vi "GeoData.vi"() -> ()   [LabVIEW 2017] (continued)
\tH1\n55474\t27053\tMinneapolis\tMN\tHennepin County\tH1\n55356\t27053\tLong lake\tMN\tHennepin County\tH1\n55404\t27053\tMinneapolis\tMN\tHennepin County\tH1\n55411\t27053\tMinneapolis\tMN\tHennepin County\tH1\n55423\t27053\tMinneapolis\tMN\tHennepin County\tH1\n55424\t27053\tMinneapolis\tMN\tHennepin County\tH1\n55429\t27053\tMinneapolis\tMN\tHennepin County\tH1\n55436\t27053\tMinneapolis\tMN\tHennepin County\tH1\n55420\t27053\tMinneapolis\tMN\tHennepin County\tH1\n55414\t27053\tMinneapolis\tMN\tHennepin County\tH1\n55416\t27053\tMinneapolis\tMN\tHennepin County\tH1\n55412\t27053\tMinneapolis\tMN\tHennepin County\tH1\n55419\t27053\tMinneapolis\tMN\tHennepin County\tH1\n55454\t27053\tMinneapolis\tMN\tHennepin County\tH1\n55442\t27053\tMinneapolis\tMN\tHennepin County\tH1\n55450\t27053\tMinneapolis\tMN\tHennepin County\tH1\n55480\t27053\tMinneapolis\tMN\tHennepin County\tH1\n55467\t27053\tMinneapolis\tMN\tHennepin County\tH1\n55305\t27053\tHopkins\tMN\tHennepin County\tH1\n55369\t27053\tOsseo\tMN\tHennepin County\tH1\n55391\t27053\tWayzata\tMN\tHennepin County\tH1\n55347\t27053\tEden prairie\tMN\tHennepin County\tH1\n55407\t27053\tMinneapolis\tMN\tHennepin County\tH1\n55357\t27053\tLoretto\tMN\tHennepin County\tH1\n55422\t27053\tMinneapolis\tMN\tHennepin County\tH1\n55427\t27053\tMinneapolis\tMN\tHennepin County\tH1\n55430\t27053\tMinneapolis\tMN\tHennepin County\tH1\n55415\t27053\tMinneapolis\tMN\tHennepin County\tH1\n55323\t27053\tCrystal bay\tMN\tHennepin County\tH1\n55488\t27053\tMinneapolis\tMN\tHennepin County\tH1\n55931\t27055\tEitzen\tMN\tHouston County\tH1\n55971\t27055\tRushford\tMN\tHouston County\tH1\n55947\t27055\tLa crescent\tMN\tHouston County\tH1\n55943\t27055\tHouston\tMN\tHouston County\tH1\n55921\t27055\tCaledonia\tMN\tHouston County\tH1\n55954\t27055\tMabel\tMN\tHouston County\tH1\n55974\t27055\tSpring grove\tMN\tHouston County\tH1\n55919\t27055\tBrownsville\tMN\tHouston County\tH1\n55941\t27055\tHokah\tMN\tHouston County\tH1\n56678\t27057\tSolway\tMN\tHubbard County\tH1\n56436\t27057\tBenedict\tMN\tHubbard County\tH1\n56464\t27057\tMenahga\tMN\tHubbard County\tH1\n56461\t27057\tLaporte\tMN\tHubbard County\tH1\n56633\t27057\tCass lake\tMN\tHubbard County\tH1\n56470\t27057\tPark rapids\tMN\tHubbard County\tH1\n56601\t27057\tBemidji\tMN\tHubbard County\tH1\n56467\t27057\tNevis\tMN\tHubbard County\tH1\n56458\t27057\tLake george\tMN\tHubbard County\tH1\n56484\t27057\tWalker\tMN\tHubbard County\tH1\n56433\t27057\tAkeley\tMN\tHubbard County\tH1\n56435\t27057\tBackus\tMN\tHubbard County\tH1\n56353\t27059\tMilaca\tMN\tIsanti County\tH1\n56358\t27059\tOgilvie\tMN\tIsanti County\tH1\n55032\t27059\tHarris\tMN\tIsanti County\tH1\n55017\t27059\tDalbo\tMN\tIsanti County\tH1\n55080\t27059\tStanchfield\tMN\tIsanti County\tH1\n55008\t27059\tCambridge\tMN\tIsanti County\tH1\n55006\t27059\tBraham\tMN\tIsanti County\tH1\n55056\t27059\tNorth branch\tMN\tIsanti County\tH1\n55070\t27059\tSaint francis\tMN\tIsanti County\tH1\n55398\t27059\tZimmerman\tMN\tIsanti County\tH1\n55029\t27059\tGrandy\tMN\tIsanti County\tH1\n55005\t27059\tBethel\tMN\tIsanti County\tH1\n55040\t27059\tIsanti\tMN\tIsanti County\tH1\n55079\t27059\tStacy\tMN\tIsanti County\tH1\n55371\t27059\tPrinceton\tMN\tIsanti County\tH1\n55771\t27061\tOrr\tMN\tItasca County\tH1\n56636\t27061\tDeer river\tMN\tItasca County\tH1\n55781\t27061\tSide lake\tMN\tItasca County\tH1\n55736\t27061\tFloodwood\tMN\tItasca County\tH1\n56630\t27061\tBlackduck\tMN\tItasca County\tH1\n56628\t27061\tBigfork\tMN\tItasca County\tH1\n56681\t27061\tSquaw lake\tMN\tItasca County\tH1\n55723\t27061\tCook\tMN\tItasca County\tH1\n55769\t27061\tNashwauk\tMN\tItasca County\tH1\n55709\t27061\tBovey\tMN\tItasca County\tH1\n56661\t27061\tNorthome\tMN\tItasca County\tH1\n56680\t27061\tSpring lake\tMN\tItasca County\tH1\n56639\t27061\tEffie\tMN\tItasca County\tH1\n55764\t27061\tMarble\tMN\tItasca County\tH1\n55753\t27061\tKeewatin\tMN\tItasca County\tH1\n55745\t27061\tGrand rapids\tMN\tItasca County\tH1\n55746\t27061\tHibbing\tMN\tItasca County\tH1\n55742\t27061\tGoodland\tMN\tItasca County\tH1\n55775\t27061\tPengilly\tMN\tItasca County\tH1\n56657\t27061\tMarcell\tMN\tItasca County\tH1\n56688\t27061\tWirt\tMN\tItasca County\tH1\n55744\t27061\tGrand rapids\tMN\tItasca County\tH1\n56659\t27061\tMax\tMN\tItasca County\tH1\n55722\t27061\tColeraine\tMN\tItasca County\tH1\n55752\t27061\tJacobson\tMN\tItasca County\tH1\n55793\t27061\tWarba\tMN\tItasca County\tH1\n56637\t27061\tTalmoon\tMN\tItasca County\tH1\n55748\t27061\tHill city\tMN\tItasca County\tH1\n55721\t27061\tCohasset\tMN\tItasca County\tH1\n55784\t27061\tSwan river\tMN\tItasca County\tH1\n55716\t27061\tCalumet\tMN\tItasca County\tH1\n56631\t27061\tBowstring\tMN\tItasca County\tH1\n55786\t27061\tTaconite\tMN\tItasca County\tH1\n56159\t27063\tMountain lake\tMN\tJackson County\tH1\n56160\t27063\tOdin\tMN\tJackson County\tH1\n56137\t27063\tHeron lake\tMN\tJackson County\tH1\n56150\t27063\tLakefield\tMN\tJackson County\tH1\n56187\t27063\tWorthington\tMN\tJackson County\tH1\n56143\t27063\tJackson\tMN\tJackson County\tH1\n56131\t27063\tFulda\tMN\tJackson County\tH1\n56119\t27063\tBrewster\tMN\tJackson County\tH1\n56167\t27063\tRound lake\tMN\tJackson County\tH1\n56111\t27063\tAlpha\tMN\tJackson County\tH1\n56101\t27063\tWindom\tMN\tJackson County\tH1\n56118\t27063\tBingham lake\tMN\tJackson County\tH1\n56161\t27063\tOkabena\tMN\tJackson County\tH1\n56127\t27063\tDunnell\tMN\tJackson County\tH1\n56353\t27065\tMilaca\tMN\tKanabec County\tH1\n56358\t27065\tOgilvie\tMN\tKanabec County\tH1\n55030\t27065\tGrasston\tMN\tKanabec County\tH1\n55037\t27065\tHinckley\tMN\tKanabec County\tH1\n56342\t27065\tIsle\tMN\tKanabec County\tH1\n55006\t27065\tBraham\tMN\tKanabec County\tH1\n55051\t27065\tMora\tMN\tKanabec County\tH1\n55007\t27065\tBrook park\tMN\tKanabec County\tH1\n55072\t27065\tSandstone\tMN\tKanabec County\tH1\n56312\t27067\tBelgrade\tMN\tKandiyohi County\tH1\n56201\t27067\tWillmar\tMN\tKandiyohi County\tH1\n56362\t27067\tPaynesville\tMN\tKandiyohi County\tH1\n56273\t27067\tNew london\tMN\tKandiyohi County\tH1\n56316\t27067\tBrooten\tMN\tKandiyohi County\tH1\n56284\t27067\tRenville\tMN\tKandiyohi County\tH1\n56289\t27067\tSunburg\tMN\tKandiyohi County\tH1\n56252\t27067\tKerkhoven\tMN\tKandiyohi County\tH1\n56281\t27067\tPrinsburg\tMN\tKandiyohi County\tH1\n56277\t27067\tOlivia\tMN\tKandiyohi County\tH1\n56288\t27067\tSpicer\tMN\tKandiyohi County\tH1\n56251\t27067\tKandiyohi\tMN\tKandiyohi County\tH1\n56216\t27067\tBlomkest\tMN\tKandiyohi County\tH1\n56253\t27067\tLake lillian\tMN\tKandiyohi County\tH1\n56243\t27067\tGrove city\tMN\tKandiyohi County\tH1\n56279\t27067\tPennock\tMN\tKandiyohi County\tH1\n56282\t27067\tRaymond\tMN\tKandiyohi County\tH1\n56222\t27067\tClara city\tMN\tKandiyohi County\tH1\n56209\t27067\tAtwater\tMN\tKandiyohi County\tH1\n56755\t27069\tSaint vincent\tMN\tKittson County\tH1\n56740\t27069\tNoyes\tMN\tKittson County\tH1\n56729\t27069\tHalma\tMN\tKittson County\tH1\n56733\t27069\tKennedy\tMN\tKittson County\tH1\n56734\t27069\tLake bronson\tMN\tKittson County\tH1\n56732\t27069\tKarlstad\tMN\tKittson County\tH1\n56731\t27069\tHumboldt\tMN\tKittson County\tH1\n56735\t27069\tLancaster\tMN\tKittson County\tH1\n56720\t27069\tDonaldson\tMN\tKittson County\tH1\n56728\t27069\tHallock\tMN\tKittson County\tH1\n55771\t27071\tOrr\tMN\tKoochiching County\tH1\n56654\t27071\tLoman\tMN\tKoochiching County\tH1\n56661\t27071\tNorthome\tMN\tKoochiching County\tH1\n56639\t27071\tEffie\tMN\tKoochiching County\tH1\n56668\t27071\tRanier\tMN\tKoochiching County\tH1\n56629\t27071\tBirchdale\tMN\tKoochiching County\tH1\n56660\t27071\tMizpah\tMN\tKoochiching County\tH1\n56653\t27071\tLittlefork\tMN\tKoochiching County\tH1\n56627\t27071\tBig falls\tMN\tKoochiching County\tH1\n56649\t27071\tInternational falls\tMN\tKoochiching County\tH1\n56679\t27071\tSouth international falls\tMN\tKoochiching County\tH1\n56623\t27071\tBaudette\tMN\tKoochiching County\tH1\n56669\t27071\tKabetogama\tMN\tKoochiching County\tH1\n56658\t27071\tMargie\tMN\tKoochiching County\tH1\n55772\t27071\tNett lake\tMN\tKoochiching County\tH1\n56223\t27073\tClarkfield\tMN\tLac qui Parle County\tH1\n56257\t27073\tMarietta\tMN\tLac qui Parle County\tH1\n56256\t27073\tMadison\tMN\tLac qui Parle County\tH1\n56278\t27073\tOrtonville\tMN\tLac qui Parle County\tH1\n56220\t27073\tCanby\tMN\tLac qui Parle County\tH1\n56265\t27073\tMontevideo\tMN\tLac qui Parle County\tH1\n56208\t27073\tAppleton\tMN\tLac qui Parle County\tH1\n56218\t27073\tBoyd\tMN\tLac qui Parle County\tH1\n56232\t27073\tDawson\tMN\tLac qui Parle County\tH1\n56276\t27073\tOdessa\tMN\tLac qui Parle County\tH1\n56212\t27073\tBellingham\tMN\tLac qui Parle County\tH1\n55614\t27075\tSilver bay\tMN\tLake County\tH1\n55616\t27075\tTwo harbors\tMN\tLake County\tH1\n55607\t27075\tIsabella\tMN\tLake County\tH1\n55731\t27075\tEly\tMN\tLake County\tH1\n55609\t27075\tKnife river\tMN\tLake County\tH1\n55602\t27075\tBrimson\tMN\tLake County\tH1\n55603\t27075\tFinland\tMN\tLake County\tH1\n55601\t27075\tBeaver bay\tMN\tLake County\tH1\n56711\t27077\tAngle inlet\tMN\tLake of the Woods County\tH1\n56623\t27077\tBaudette\tMN\tLake of the Woods County\tH1\n56673\t27077\tRoosevelt\tMN\tLake of the Woods County\tH1\n56741\t27077\tOak island\tMN\tLake of the Woods County\tH1\n56686\t27077\tWilliams\tMN\tLake of the Woods County\tH1\n56096\t27079\tWaterville\tMN\tLe Sueur County\tH1\n56052\t27079\tKilkenny\tMN\tLe Sueur County\tH1\n56050\t27079\tKasota\tMN\tLe Sueur County\tH1\n56071\t27079\tNew prague\tMN\tLe Sueur County\tH1\n56063\t27079\tMadison lake\tMN\tLe Sueur County\tH1\n56069\t27079\tMontgomery\tMN\tLe Sueur County\tH1\n56011\t27079\tBelle plaine\tMN\tLe Sueur County\tH1\n56058\t27079\tLe sueur\tMN\tLe Sueur County\tH1\n56057\t27079\tLe center\tMN\tLe Sueur County\tH1\n56028\t27079\tElysian\tMN\tLe Sueur County\tH1\n56082\t27079\tSaint peter\tMN\tLe Sueur County\tH1\n56017\t27079\tCleveland\tMN\tLe Sueur County\tH1\n56044\t27079\tHenderson\tMN\tLe Sueur County\tH1\n56264\t27081\tMinneota\tMN\tLincoln County\tH1\n56291\t27081\tTaunton\tMN\tLincoln County\tH1\n56170\t27081\tRuthton\tMN\tLincoln County\tH1\n56142\t27081\tIvanhoe\tMN\tLincoln County\tH1\n56178\t27081\tTyler\tMN\tLincoln County\tH1\n56220\t27081\tCanby\tMN\tLincoln County\tH1\n56136\t27081\tHendricks\tMN\tLincoln County\tH1\n56164\t27081\tPipestone\tMN\tLincoln County\tH1\n56113\t27081\tArco\tMN\tLincoln County\tH1\n56149\t27081\tLake benton\tMN\tLincoln County\tH1\n56280\t27081\tPorter\tMN\tLincoln County\tH1\n56264\t27083\tMinneota\tMN\tLyon County\tH1\n56291\t27083\tTaunton\tMN\tLyon County\tH1\n56170\t27083\tRuthton\tMN\tLyon County\tH1\n56157\t27083\tLynd\tMN\tLyon County\tH1\n56115\t27083\tBalaton\tMN\tLyon County\tH1\n56175\t27083\tTracy\tMN\tLyon County\tH1\n56178\t27083\tTyler\tMN\tLyon County\tH1\n56263\t27083\tMilroy\tMN\tLyon County\tH1\n56220\t27083\tCanby\tMN\tLyon County\tH1\n56258\t27083\tMarshall\tMN\tLyon County\tH1\n56297\t27083\tWood lake\tMN\tLyon County\tH1\n56229\t27083\tCottonwood\tMN\tLyon County\tH1\n56239\t27083\tGhent\tMN\tLyon County\tH1\n56113\t27083\tArco\tMN\tLyon County\tH1\n56169\t27083\tRussell\tMN\tLyon County\tH1\n56132\t27083\tGarvin\tMN\tLyon County\tH1\n56280\t27083\tPorter\tMN\tLyon County\tH1\n55312\t27085\tBrownton\tMN\tMcLeod County\tH1\n55370\t27085\tPlato\tMN\tMcLeod County\tH1\n55355\t27085\tLitchfield\tMN\tMcLeod County\tH1\n55368\t27085\tNorwood young america\tMN\tMcLeod County\tH1\n55339\t27085\tHamburg\tMN\tMcLeod County\tH1\n55350\t27085\tHutchinson\tMN\tMcLeod County\tH1\n55338\t27085\tGreen isle\tMN\tMcLeod County\tH1\n55381\t27085\tSilver lake\tMN\tMcLeod County\tH1\n55335\t27085\tGibbon\tMN\tMcLeod County\tH1\n55336\t27085\tGlencoe\tMN\tMcLeod County\tH1\n55354\t27085\tLester prairie\tMN\tMcLeod County\tH1\n55367\t27085\tNew germany\tMN\tMcLeod County\tH1\n55396\t27085\tWinthrop\tMN\tMcLeod County\tH1\n55385\t27085\tStewart\tMN\tMcLeod County\tH1\n55397\t27085\tYoung america\tMN\tMcLeod County\tH1\n55395\t27085\tWinsted\tMN\tMcLeod County\tH1\n56651\t27087\tLengby\tMN\tMahnomen County\tH1\n56621\t27087\tBagley\tMN\tMahnomen County\tH1\n56540\t27087\tFertile\tMN\tMahnomen County\tH1\n56589\t27087\tWaubun\tMN\tMahnomen County\tH1\n56592\t27087\tWinger\tMN\tMahnomen County\tH1\n56566\t27087\tNaytahwaush\tMN\tMahnomen County\tH1\n56557\t27087\tMahnomen\tMN\tMahnomen County\tH1\n56542\t27087\tFosston\tMN\tMahnomen County\tH1\n56516\t27087\tBejou\tMN\tMahnomen County\tH1\n56727\t27089\tGrygla\tMN\tMarshall County\tH1\n56744\t27089\tOslo\tMN\tMarshall County\tH1\n56757\t27089\tStephen\tMN\tMarshall County\tH1\n56762\t27089\tWarren\tMN\tMarshall County\tH1\n56724\t27089\tGatzke\tMN\tMarshall County\tH1\n56758\t27089\tStrandquist\tMN\tMarshall County\tH1\n56760\t27089\tViking\tMN\tMarshall County\tH1\n56738\t27089\tNewfolden\tMN\tMarshall County\tH1\n56732\t27089\tKarlstad\tMN\tMarshall County\tH1\n56759\t27089\tStrathcona\tMN\tMarshall County\tH1\n56710\t27089\tAlvarado\tMN\tMarshall County\tH1\n56701\t27089\tThief river falls\tMN\tMarshall County\tH1\n56713\t27089\tArgyle\tMN\tMarshall County\tH1\n56725\t27089\tGoodridge\tMN\tMarshall County\tH1\n56737\t27089\tMiddle river\tMN\tMarshall County\tH1\n56098\t27091\tWinnebago\tMN\tMartin County\tH1\n56027\t27091\tElmore\tMN\tMartin County\tH1\n56162\t27091\tOrmsby\tMN\tMartin County\tH1\n56160\t27091\tOdin\tMN\tMartin County\tH1\n56031\t27091\tFairmont\tMN\tMartin County\tH1\n56181\t27091\tWelcome\tMN\tMartin County\tH1\n56075\t27091\tNorthrop\tMN\tMartin County\tH1\n56176\t27091\tTrimont\tMN\tMartin County\tH1\n56171\t27091\tSherburn\tMN\tMartin County\tH1\n56121\t27091\tCeylon\tMN\tMartin County\tH1\n56013\t27091\tBlue earth\tMN\tMartin County\tH1\n56111\t27091\tAlpha\tMN\tMartin County\tH1\n56039\t27091\tGranada\tMN\tMartin County\tH1\n56088\t27091\tTruman\tMN\tMartin County\tH1\n56127\t27091\tDunnell\tMN\tMartin County\tH1\n55353\t27093\tKimball\tMN\tMeeker County\tH1\n56362\t27093\tPaynesville\tMN\tMeeker County\tH1\n56228\t27093\tCosmos\tMN\tMeeker County\tH1\n55324\t27093\tDarwin\tMN\tMeeker County\tH1\n55355\t27093\tLitchfield\tMN\tMeeker County\tH1\n55389\t27093\tWatkins\tMN\tMeeker County\tH1\n55350\t27093\tHutchinson\tMN\tMeeker County\tH1\n55321\t27093\tCokato\tMN\tMeeker County\tH1\n55342\t27093\tHector\tMN\tMeeker County\tH1\n55382\t27093\tSouth haven\tMN\tMeeker County\tH1\n55329\t27093\tEden valley\tMN\tMeeker County\tH1\n56243\t27093\tGrove city\tMN\tMeeker County\tH1\n55325\t27093\tDassel\tMN\tMeeker County\tH1\n56209\t27093\tAtwater\tMN\tMeeker County\tH1\n56353\t27095\tMilaca\tMN\tMille Lacs County\tH1\n56358\t27095\tOgilvie\tMN\tMille Lacs County\tH1\n56363\t27095\tPease\tMN\tMille Lacs County\tH1\n56313\t27095\tBock\tMN\tMille Lacs County\tH1\n56330\t27095\tForeston\tMN\tMille Lacs County\tH1\n56342\t27095\tIsle\tMN\tMille Lacs County\tH1\n56338\t27095\tHillman\tMN\tMille Lacs County\tH1\n56359\t27095\tOnamia\tMN\tMille Lacs County\tH1\n56450\t27095\tGarrison\tMN\tMille Lacs County\tH1\n55371\t27095\tPrinceton\tMN\tMille Lacs County\tH1\n56357\t27095\tOak park\tMN\tMille Lacs County\tH1\n56386\t27095\tWahkon\tMN\tMille Lacs County\tH1\n56353\t27097\tMilaca\tMN\tMorrison County\tH1\n56364\t27097\tPierz\tMN\tMorrison County\tH1\n56347\t27097\tLong prairie\tMN\tMorrison County\tH1\n56307\t27097\tAlbany\tMN\tMorrison County\tH1\n56345\t27097\tLittle falls\tMN\tMorrison County\tH1\n56336\t27097\tGrey eagle\tMN\tMorrison County\tH1\n56443\t27097\tCushing\tMN\tMorrison County\tH1\n56314\t27097\tBowlus\tMN\tMorrison County\tH1\n56338\t27097\tHillman\tMN\tMorrison County\tH1\n56367\t27097\tRice\tMN\tMorrison County\tH1\n56331\t27097\tFreeport\tMN\tMorrison County\tH1\n56328\t27097\tFlensburg\tMN\tMorrison County\tH1\n56384\t27097\tUpsala\tMN\tMorrison County\tH1\n56344\t27097\tLastrup\tMN\tMorrison County\tH1\n56318\t27097\tBurtrum\tMN\tMorrison County\tH1\n56359\t27097\tOnamia\tMN\tMorrison County\tH1\n56473\t27097\tPillager\tMN\tMorrison County\tH1\n56449\t27097\tFort ripley\tMN\tMorrison County\tH1\n56466\t27097\tMotley\tMN\tMorrison County\tH1\n56373\t27097\tRoyalton\tMN\tMorrison County\tH1\n56340\t27097\tHoldingford\tMN\tMorrison County\tH1\n56475\t27097\tRandall\tMN\tMorrison County\tH1\n56329\t27097\tFoley\tMN\tMorrison County\tH1\n56382\t27097\tSwanville\tMN\tMorrison County\tH1\n55926\t27099\tDexter\tMN\tMower County\tH1\n55936\t27099\tGrand meadow\tMN\tMower County\tH1\n55975\t27099\tSpring valley\tMN\tMower County\tH1\n55918\t27099\tBrownsdale\tMN\tMower County\tH1\n55951\t27099\tLe roy\tMN\tMower County\tH1\n55917\t27099\tBlooming prairie\tMN\tMower County\tH1\n55909\t27099\tAdams\tMN\tMower County\tH1\n55967\t27099\tRacine\tMN\tMower County\tH1\n55933\t27099\tElkton\tMN\tMower County\tH1\n55973\t27099\tSargeant\tMN\tMower County\tH1\n55940\t27099\tHayfield\tMN\tMower County\tH1\n55976\t27099\tStewartville\tMN\tMower County\tH1\n55970\t27099\tRose creek\tMN\tMower County\tH1\n55950\t27099\tLansing\tMN\tMower County\tH1\n55912\t27099\tAustin\tMN\tMower County\tH1\n55961\t27099\tOstrander\tMN\tMower County\tH1\n55982\t27099\tWaltham\tMN\tMower County\tH1\n55953\t27099\tLyle\tMN\tMower County\tH1\n55977\t27099\tTaopi\tMN\tMower County\tH1\n56180\t27101\tWalnut grove\tMN\tMurray County\tH1\n56172\t27101\tSlayton\tMN\tMurray County\tH1\n56170\t27101\tRuthton\tMN\tMurray County\tH1\n56141\t27101\tIona\tMN\tMurray County\tH1\n56125\t27101\tDovray\tMN\tMurray County\tH1\n56115\t27101\tBalaton\tMN\tMurray County\tH1\n56122\t27101\tChandler\tMN\tMurray County\tH1\n56151\t27101\tLake wilson\tMN\tMurray County\tH1\n56175\t27101\tTracy\tMN\tMurray County\tH1\n56114\t27101\tAvoca\tMN\tMurray County\tH1\n56131\t27101\tFulda\tMN\tMurray County\tH1\n56186\t27101\tWoodstock\tMN\tMurray County\tH1\n56128\t27101\tEdgerton\tMN\tMurray County\tH1\n56183\t27101\tWestbrook\tMN\tMurray County\tH1\n56123\t27101\tCurrie\tMN\tMurray County\tH1\n56132\t27101\tGarvin\tMN\tMurray County\tH1\n56149\t27101\tLake benton\tMN\tMurray County\tH1\n56054\t27103\tLafayette\tMN\tNicollet County\tH1\n55335\t27103\tGibbon\tMN\tNicollet County\tH1\n56001\t27103\tMankato\tMN\tNicollet County\tH1\n56058\t27103\tLe sueur\tMN\tNicollet County\tH1\n56003\t27103\tMankato\tMN\tNicollet County\tH1\n56073\t27103\tNew ulm\tMN\tNicollet County\tH1\n56074\t27103\tNicollet\tMN\tNicollet County\tH1\n55334\t27103\tGaylord\tMN\tNicollet County\tH1\n55332\t27103\tFairfax\tMN\tNicollet County\tH1\n56082\t27103\tSaint peter\tMN\tNicollet County\tH1\n56021\t27103\tCourtland\tMN\tNicollet County\tH1\n56158\t27105\tMagnolia\tMN\tNobles County\tH1\n56141\t27105\tIona\tMN\tNobles County\tH1\n56122\t27105\tChandler\tMN\tNobles County\tH1\n56137\t27105\tHeron lake\tMN\tNobles County\tH1\n56153\t27105\tLeota\tMN\tNobles County\tH1\n56110\t27105\tAdrian\tMN\tNobles County\tH1\n56187\t27105\tWorthington\tMN\tNobles County\tH1\n56131\t27105\tFulda\tMN\tNobles County\tH1\n56119\t27105\tBrewster\tMN\tNobles County\tH1\n56185\t27105\tWilmont\tMN\tNobles County\tH1\n56167\t27105\tRound lake\tMN\tNobles County\tH1\n56128\t27105\tEdgerton\tMN\tNobles County\tH1\n56165\t27105\tReading\tMN\tNobles County\tH1\n56117\t27105\tBigelow\tMN\tNobles County\tH1\n56129\t27105\tEllsworth\tMN\tNobles County\tH1\n56155\t27105\tLismore\tMN\tNobles County\tH1\n56168\t27105\tRushmore\tMN\tNobles County\tH1\n56147\t27105\tKenneth\tMN\tNobles County\tH1\n56584\t27107\tTwin valley\tMN\tNorman County\tH1\n56545\t27107\tGary\tMN\tNorman County\tH1\n56550\t27107\tHendrum\tMN\tNorman County\tH1\n56585\t27107\tUlen\tMN\tNorman County\tH1\n56541\t27107\tFlom\tMN\tNorman County\tH1\n56510\t27107\tAda\tMN\tNorman County\tH1\n56581\t27107\tShelly\tMN\tNorman County\tH1\n56574\t27107\tPerley\tMN\tNorman County\tH1\n56540\t27107\tFertile\tMN\tNorman County\tH1\n56589\t27107\tWaubun\tMN\tNorman County\tH1\n56546\t27107\tGeorgetown\tMN\tNorman County\tH1\n56519\t27107\tBorup\tMN\tNorman County\tH1\n56557\t27107\tMahnomen\tMN\tNorman County\tH1\n56568\t27107\tNielsville\tMN\tNorman County\tH1\n56548\t27107\tHalstad\tMN\tNorman County\tH1\n56516\t27107\tBejou\tMN\tNorman County\tH1\n55906\t27109\tRochester\tMN\tOlmsted County\tH1\n55960\t27109\tOronoco\tMN\tOlmsted County\tH1\n55944\t27109\tKasson\tMN\tOlmsted County\tH1\n55903\t27109\tRochester\tMN\tOlmsted County\tH1\n55901\t27109\tRochester\tMN\tOlmsted County\tH1\n55904\t27109\tRochester\tMN\tOlmsted County\tH1\n55923\t27109\tChatfield\tMN\tOlmsted County\tH1\n55905\t27109\tRochester\tMN\tOlmsted County\tH1\n55934\t27109\tEyota\tMN\tOlmsted County\tH1\n55955\t27109\tMantorville\tMN\tOlmsted County\tH1\n55920\t27109\tByron\tMN\tOlmsted County\tH1\n55972\t27109\tSaint charles\tMN\tOlmsted County\tH1\n55991\t27109\tZumbro falls\tMN\tOlmsted County\tH1\n55932\t27109\tElgin\tMN\tOlmsted County\tH1\n55973\t27109\tSargeant\tMN\tOlmsted County\tH1\n55902\t27109\tRochester\tMN\tOlmsted County\tH1\n55956\t27109\tMazeppa\tMN\tOlmsted County\tH1\n55940\t27109\tHayfield\tMN\tOlmsted County\tH1\n55964\t27109\tPlainview\tMN\tOlmsted County\tH1\n55963\t27109\tPine island\tMN\tOlmsted County\tH1\n55976\t27109\tStewartville\tMN\tOlmsted County\tH1\n55929\t27109\tDover\tMN\tOlmsted County\tH1\n56527\t27111\tDeer creek\tMN\tOtter Tail County\tH1\n56573\t27111\tPerham\tMN\tOtter Tail County\tH1\n56531\t27111\tElbow lake\tMN\tOtter Tail County\tH1\n56534\t27111\tErhard\tMN\tOtter Tail County\tH1\n56551\t27111\tHenning\tMN\tOtter Tail County\tH1\n56464\t27111\tMenahga\tMN\tOtter Tail County\tH1\n56315\t27111\tBrandon\tMN\tOtter Tail County\tH1\n56437\t27111\tBertha\tMN\tOtter Tail County\tH1\n56587\t27111\tVergas\tMN\tOtter Tail County\tH1\n56588\t27111\tVining\tMN\tOtter Tail County\tH1\n56567\t27111\tNew york mills\tMN\tOtter Tail County\tH1\n56528\t27111\tDent\tMN\tOtter Tail County\tH1\n56524\t27111\tClitherall\tMN\tOtter Tail County\tH1\n56477\t27111\tSebeka\tMN\tOtter Tail County\tH1\n56453\t27111\tHewitt\tMN\tOtter Tail County\tH1\n56590\t27111\tWendell\tMN\tOtter Tail County\tH1\n56309\t27111\tAshby\tMN\tOtter Tail County\tH1\n56361\t27111\tParkers prairie\tMN\tOtter Tail County\tH1\n56515\t27111\tBattle lake\tMN\tOtter Tail County\tH1\n56326\t27111\tEvansville\tMN\tOtter Tail County\tH1\n56533\t27111\tElizabeth\tMN\tOtter Tail County\tH1\n56579\t27111\tRothsay\tMN\tOtter Tail County\tH1\n56583\t27111\tTintah\tMN\tOtter Tail County\tH1\n56522\t27111\tCampbell\tMN\tOtter Tail County\tH1\n56324\t27111\tDalton\tMN\tOtter Tail County\tH1\n56514\t27111\tBarnesville\tMN\tOtter Tail County\tH1\n56572\t27111\tPelican rapids\tMN\tOtter Tail County\tH1\n56482\t27111\tWadena\tMN\tOtter Tail County\tH1\n56571\t27111\tOttertail\tMN\tOtter Tail County\tH1\n56354\t27111\tMiltona\tMN\tOtter Tail County\tH1\n56501\t27111\tDetroit lakes\tMN\tOtter Tail County\tH1\n56576\t27111\tRichville\tMN\tOtter Tail County\tH1\n56446\t27111\tEagle bend\tMN\tOtter Tail County\tH1\n56544\t27111\tFrazee\tMN\tOtter Tail County\tH1\n56537\t27111\tFergus falls\tMN\tOtter Tail County\tH1\n56586\t27111\tUnderwood\tMN\tOtter Tail County\tH1\n56518\t27111\tBluffton\tMN\tOtter Tail County\tH1\n56748\t27113\tPlummer\tMN\tPennington County\tH1\n56760\t27113\tViking\tMN\tPennington County\tH1\n56754\t27113\tSaint hilaire\tMN\tPennington County\tH1\n56750\t27113\tRed lake falls\tMN\tPennington County\tH1\n56701\t27113\tThief river falls\tMN\tPennington County\tH1\n56725\t27113\tGoodridge\tMN\tPennington County\tH1\n55063\t27115\tPine city\tMN\tPine County\tH1\n55069\t27115\tRush city\tMN\tPine County\tH1\n55036\t27115\tHenriette\tMN\tPine County\tH1\n55735\t27115\tFinlayson\tMN\tPine County\tH1\n55030\t27115\tGrasston\tMN\tPine County\tH1\n55037\t27115\tHinckley\tMN\tPine County\tH1\n55795\t27115\tWillow river\tMN\tPine County\tH1\n55749\t27115\tHolyoke\tMN\tPine County\tH1\n55756\t27115\tKerrick\tMN\tPine County\tH1\n55006\t27115\tBraham\tMN\tPine County\tH1\n56350\t27115\tMc grath\tMN\tPine County\tH1\n55051\t27115\tMora\tMN\tPine County\tH1\n55712\t27115\tBruno\tMN\tPine County\tH1\n55767\t27115\tMoose lake\tMN\tPine County\tH1\n55007\t27115\tBrook park\tMN\tPine County\tH1\n55072\t27115\tSandstone\tMN\tPine County\tH1\n55704\t27115\tAskov\tMN\tPine County\tH1\n55783\t27115\tSturgeon lake\tMN\tPine County\tH1\n56170\t27117\tRuthton\tMN\tPipestone County\tH1\n56164\t27117\tPipestone\tMN\tPipestone County\tH1\n56186\t27117\tWoodstock\tMN\tPipestone County\tH1\n56128\t27117\tEdgerton\tMN\tPipestone County\tH1\n56139\t27117\tHolland\tMN\tPipestone County\tH1\n56144\t27117\tJasper\tMN\tPipestone County\tH1\n56156\t27117\tLuverne\tMN\tPipestone County\tH1\n56149\t27117\tLake benton\tMN\tPipestone County\tH1\n56721\t27119\tEast grand forks\tMN\tPolk County\tH1\n56723\t27119\tFisher\tMN\tPolk County\tH1\n56556\t27119\tMcintosh\tMN\tPolk County\tH1\n56523\t27119\tClimax\tMN\tPolk County\tH1\n56744\t27119\tOslo\tMN\tPolk County\tH1\n56742\t27119\tOklee\tMN\tPolk County\tH1\n56651\t27119\tLengby\tMN\tPolk County\tH1\n56716\t27119\tCrookston\tMN\tPolk County\tH1\n56762\t27119\tWarren\tMN\tPolk County\tH1\n56621\t27119\tBagley\tMN\tPolk County\tH1\n56535\t27119\tErskine\tMN\tPolk County\tH1\n56722\t27119\tEuclid\tMN\tPolk County\tH1\n56540\t27119\tFertile\tMN\tPolk County\tH1\n56684\t27119\tTrail\tMN\tPolk County\tH1\n56592\t27119\tWinger\tMN\tPolk County\tH1\n56646\t27119\tGully\tMN\tPolk County\tH1\n56644\t27119\tGonvick\tMN\tPolk County\tH1\n56568\t27119\tNielsville\tMN\tPolk County\tH1\n56710\t27119\tAlvarado\tMN\tPolk County\tH1\n56542\t27119\tFosston\tMN\tPolk County\tH1\n56750\t27119\tRed lake falls\tMN\tPolk County\tH1\n56517\t27119\tBeltrami\tMN\tPolk County\tH1\n56736\t27119\tMentor\tMN\tPolk County\tH1\n56226\t27121\tClontarf\tMN\tPope County\tH1\n56323\t27121\tCyrus\tMN\tPope County\tH1\n56316\t27121\tBrooten\tMN\tPope County\tH1\n56343\t27121\tKensington\tMN\tPope County\tH1\n56349\t27121\tLowry\tMN\tPope County\tH1\n56289\t27121\tSunburg\tMN\tPope County\tH1\n56334\t27121\tGlenwood\tMN\tPope County\tH1\n56308\t27121\tAlexandria\tMN\tPope County\tH1\n56360\t27121\tOsakis\tMN\tPope County\tH1\n56378\t27121\tSauk centre\tMN\tPope County\tH1\n56215\t27121\tBenson\tMN\tPope County\tH1\n56381\t27121\tStarbuck\tMN\tPope County\tH1\n56327\t27121\tFarwell\tMN\tPope County\tH1\n56244\t27121\tHancock\tMN\tPope County\tH1\n56385\t27121\tVillard\tMN\tPope County\tH1\n55106\t27123\tSaint paul\tMN\tRamsey County\tH1\n55107\t27123\tSaint paul\tMN\tRamsey County\tH1\n55113\t27123\tSaint paul\tMN\tRamsey County\tH1\n55117\t27123\tSaint paul\tMN\tRamsey County\tH1\n55126\t27123\tSaint paul\tMN\tRamsey County\tH1\n55102\t27123\tSaint paul\tMN\tRamsey County\tH1\n55105\t27123\tSaint paul\tMN\tRamsey County\tH1\n55112\t27123\tSaint paul\tMN\tRamsey County\tH1\n55119\t27123\tSaint paul\tMN\tRamsey County\tH1\n55418\t27123\tMinneapolis\tMN\tRamsey County\tH1\n55104\t27123\tSaint paul\tMN\tRamsey County\tH1\n55108\t27123\tSaint paul\tMN\tRamsey County\tH1\n55114\t27123\tSaint paul\tMN\tRamsey County\tH1\n55118\t27123\tSaint paul\tMN\tRamsey County\tH1\n55127\t27123\tSaint paul\tMN\tRamsey County\tH1\n55449\t27123\tMinneapolis\tMN\tRamsey County\tH1\n55155\t27123\tSaint paul\tMN\tRamsey County\tH1\n55109\t27123\tSaint paul\tMN\tRamsey County\tH1\n55125\t27123\tSaint paul\tMN\tRamsey County\tH1\n55432\t27123\tMinneapolis\tMN\tRamsey County\tH1\n55146\t27123\tSaint paul\tMN\tRamsey County\tH1\n55421\t27123\tMinneapolis\tMN\tRamsey County\tH1\n55101\t27123\tSaint paul\tMN\tRamsey County\tH1\n55103\t27123\tSaint paul\tMN\tRamsey County\tH1\n55130\t27123\tSaint paul\tMN\tRamsey County\tH1\n55144\t27123\tSaint paul\tMN\tRamsey County\tH1\n55110\t27123\tSaint paul\tMN\tRamsey County\tH1\n55116\t27123\tSaint paul\tMN\tRamsey County\tH1\n55128\t27123\tSaint paul\tMN\tRamsey County\tH1\n56742\t27125\tOklee\tMN\tRed Lake County\tH1\n56716\t27125\tCrookston\tMN\tRed Lake County\tH1\n56748\t27125\tPlummer\tMN\tRed Lake County\tH1\n56535\t27125\tErskine\tMN\tRed Lake County\tH1\n56754\t27125\tSaint hilaire\tMN\tRed Lake County\tH1\n56715\t27125\tBrooks\tMN\tRed Lake County\tH1\n56750\t27125\tRed lake falls\tMN\tRed Lake County\tH1\n56736\t27125\tMentor\tMN\tRed Lake County\tH1\n56180\t27127\tWalnut grove\tMN\tRedwood County\tH1\n55333\t27127\tFranklin\tMN\tRedwood County\tH1\n56255\t27127\tLucan\tMN\tRedwood County\tH1\n56166\t27127\tRevere\tMN\tRedwood County\tH1\n56284\t27127\tRenville\tMN\tRedwood County\tH1\n56175\t27127\tTracy\tMN\tRedwood County\tH1\n56263\t27127\tMilroy\tMN\tRedwood County\tH1\n56266\t27127\tMorgan\tMN\tRedwood County\tH1\n56294\t27127\tWanda\tMN\tRedwood County\tH1\n56283\t27127\tRedwood falls\tMN\tRedwood County\tH1\n56258\t27127\tMarshall\tMN\tRedwood County\tH1\n56292\t27127\tVesta\tMN\tRedwood County\tH1\n56224\t27127\tClements\tMN\tRedwood County\tH1\n56214\t27127\tBelview\tMN\tRedwood County\tH1\n56085\t27127\tSleepy eye\tMN\tRedwood County\tH1\n56152\t27127\tLamberton\tMN\tRedwood County\tH1\n56297\t27127\tWood lake\tMN\tRedwood County\tH1\n56270\t27127\tMorton\tMN\tRedwood County\tH1\n56087\t27127\tSpringfield\tMN\tRedwood County\tH1\n56287\t27127\tSeaforth\tMN\tRedwood County\tH1\n56237\t27127\tEcho\tMN\tRedwood County\tH1\n56083\t27127\tSanborn\tMN\tRedwood County\tH1\n56293\t27127\tWabasso\tMN\tRedwood County\tH1\n55310\t27129\tBird island\tMN\tRenville County\tH1\n55333\t27129\tFranklin\tMN\tRenville County\tH1\n56228\t27129\tCosmos\tMN\tRenville County\tH1\n56241\t27129\tGranite falls\tMN\tRenville County\tH1\n56284\t27129\tRenville\tMN\tRenville County\tH1\n55350\t27129\tHutchinson\tMN\tRenville County\tH1\n55342\t27129\tHector\tMN\tRenville County\tH1\n56277\t27129\tOlivia\tMN\tRenville County\tH1\n56283\t27129\tRedwood falls\tMN\tRenville County\tH1\n56260\t27129\tMaynard\tMN\tRenville County\tH1\n56285\t27129\tSacred heart\tMN\tRenville County\tH1\n56270\t27129\tMorton\tMN\tRenville County\tH1\n56230\t27129\tDanube\tMN\tRenville County\tH1\n55385\t27129\tStewart\tMN\tRenville County\tH1\n55332\t27129\tFairfax\tMN\tRenville County\tH1\n55314\t27129\tBuffalo lake\tMN\tRenville County\tH1\n56096\t27131\tWaterville\tMN\tRice County\tH1\n55049\t27131\tMedford\tMN\tRice County\tH1\n55946\t27131\tKenyon\tMN\tRice County\tH1\n56052\t27131\tKilkenny\tMN\tRice County\tH1\n55057\t27131\tNorthfield\tMN\tRice County\tH1\n55020\t27131\tElko new market\tMN\tRice County\tH1\n55046\t27131\tLonsdale\tMN\tRice County\tH1\n56071\t27131\tNew prague\tMN\tRice County\tH1\n55019\t27131\tDundas\tMN\tRice County\tH1\n56069\t27131\tMontgomery\tMN\tRice County\tH1\n55088\t27131\tWebster\tMN\tRice County\tH1\n55021\t27131\tFaribault\tMN\tRice County\tH1\n55018\t27131\tDennison\tMN\tRice County\tH1\n55087\t27131\tWarsaw\tMN\tRice County\tH1\n55053\t27131\tNerstrand\tMN\tRice County\tH1\n55052\t27131\tMorristown\tMN\tRice County\tH1\n56158\t27133\tMagnolia\tMN\tRock County\tH1\n56173\t27133\tSteen\tMN\tRock County\tH1\n56146\t27133\tKanaranzi\tMN\tRock County\tH1\n56134\t27133\tHardwick\tMN\tRock County\tH1\n56116\t27133\tBeaver creek\tMN\tRock County\tH1\n56164\t27133\tPipestone\tMN\tRock County\tH1\n56128\t27133\tEdgerton\tMN\tRock County\tH1\n56129\t27133\tEllsworth\tMN\tRock County\tH1\n56138\t27133\tHills\tMN\tRock County\tH1\n56144\t27133\tJasper\tMN\tRock County\tH1\n56156\t27133\tLuverne\tMN\tRock County\tH1\n56147\t27133\tKenneth\tMN\tRock County\tH1\n56726\t27135\tGreenbush\tMN\tRoseau County\tH1\n56732\t27135\tKarlstad\tMN\tRoseau County\tH1\n56761\t27135\tWannaska\tMN\tRoseau County\tH1\n56714\t27135\tBadger\tMN\tRoseau County\tH1\n56763\t27135\tWarroad\tMN\tRoseau County\tH1\n56759\t27135\tStrathcona\tMN\tRoseau County\tH1\n56756\t27135\tSalol\tMN\tRoseau County\tH1\n56735\t27135\tLancaster\tMN\tRoseau County\tH1\n56673\t27135\tRoosevelt\tMN\tRoseau County\tH1\n56751\t27135\tRoseau\tMN\tRoseau County\tH1\n55765\t27137\tMeadowlands\tMN\tSt. Louis County\tH1\n55719\t27137\tChisholm\tMN\tSt. Louis County\tH1\n55798\t27137\tWright\tMN\tSt. Louis County\tH1\n55771\t27137\tOrr\tMN\tSt. Louis County\tH1\n55732\t27137\tEmbarrass\tMN\tSt. Louis County\tH1\n55781\t27137\tSide lake\tMN\tSt. Louis County\tH1\n55763\t27137\tMakinen\tMN\tSt. Louis County\tH1\n55807\t27137\tDuluth\tMN\tSt. Louis County\tH1\n55616\t27137\tTwo harbors\tMN\tSt. Louis County\tH1\n55803\t27137\tDuluth\tMN\tSt. Louis County\tH1\n55736\t27137\tFloodwood\tMN\tSt. Louis County\tH1\n55750\t27137\tHoyt lakes\tMN\tSt. Louis County\tH1\n55738\t27137\tForbes\tMN\tSt. Louis County\tH1\n55725\t27137\tCrane lake\tMN\tSt. Louis County\tH1\n55805\t27137\tDuluth\tMN\tSt. Louis County\tH1\n55720\t27137\tCloquet\tMN\tSt. Louis County\tH1\n55723\t27137\tCook\tMN\tSt. Louis County\tH1\n55741\t27137\tGilbert\tMN\tSt. Louis County\tH1\n55769\t27137\tNashwauk\tMN\tSt. Louis County\tH1\n55705\t27137\tAurora\tMN\tSt. Louis County\tH1\n55790\t27137\tTower\tMN\tSt. Louis County\tH1\n55702\t27137\tAlborn\tMN\tSt. Louis County\tH1\n55758\t27137\tKinney\tMN\tSt. Louis County\tH1\n55808\t27137\tDuluth\tMN\tSt. Louis County\tH1\n55810\t27137\tDuluth\tMN\tSt. Louis County\tH1\n55710\t27137\tBritt\tMN\tSt. Louis County\tH1\n55746\t27137\tHibbing\tMN\tSt. Louis County\tH1\n55733\t27137\tEsko\tMN\tSt. Louis County\tH1\n55792\t27137\tVirginia\tMN\tSt. Louis County\tH1\n55811\t27137\tDuluth\tMN\tSt. Louis County\tH1\n55731\t27137\tEly\tMN\tSt. Louis County\tH1\n55734\t27137\tEveleth\tMN\tSt. Louis County\tH1\n55717\t27137\tCanyon\tMN\tSt. Louis County\tH1\n55713\t27137\tBuhl\tMN\tSt. Louis County\tH1\n55806\t27137\tDuluth\tMN\tSt. Louis County\tH1\n55751\t27137\tIron\tMN\tSt. Louis County\tH1\n55768\t27137\tMountain iron\tMN\tSt. Louis County\tH1\n55791\t27137\tTwig\tMN\tSt. Louis County\tH1\n55796\t27137\tWinton\tMN\tSt. Louis County\tH1\n55812\t27137\tDuluth\tMN\tSt. Louis County\tH1\n55724\t27137\tCotton\tMN\tSt. Louis County\tH1\n56669\t27137\tKabetogama\tMN\tSt. Louis County\tH1\n55602\t27137\tBrimson\tMN\tSt. Louis County\tH1\n55804\t27137\tDuluth\tMN\tSt. Louis County\tH1\n55779\t27137\tSaginaw\tMN\tSt. Louis County\tH1\n55802\t27137\tDuluth\tMN\tSt. Louis County\tH1\n55816\t27137\tDuluth\tMN\tSt. Louis County\tH1\n55708\t27137\tBiwabik\tMN\tSt. Louis County\tH1\n55706\t27137\tBabbitt\tMN\tSt. Louis County\tH1\n55703\t27137\tAngora\tMN\tSt. Louis County\tH1\n55711\t27137\tBrookston\tMN\tSt. Louis County\tH1\n55782\t27137\tSoudan\tMN\tSt. Louis County\tH1\n55337\t27139\tBurnsville\tMN\tScott County\tH1\n55352\t27139\tJordan\tMN\tScott County\tH1\n55378\t27139\tSavage\tMN\tScott County\tH1\n55020\t27139\tElko new market\tMN\tScott County\tH1\n56071\t27139\tNew prague\tMN\tScott County\tH1\n55379\t27139\tShakopee\tMN\tScott County\tH1\n56011\t27139\tBelle plaine\tMN\tScott County\tH1\n55044\t27139\tLakeville\tMN\tScott County\tH1\n55088\t27139\tWebster\tMN\tScott County\tH1\n55054\t27139\tElko new market\tMN\tScott County\tH1\n55372\t27139\tPrior lake\tMN\tScott County\tH1\n56044\t27139\tHenderson\tMN\tScott County\tH1\n56379\t27141\tSauk rapids\tMN\tSherburne County\tH1\n55308\t27141\tBecker\tMN\tSherburne County\tH1\n55330\t27141\tElk river\tMN\tSherburne County\tH1\n55309\t27141\tBig lake\tMN\tSherburne County\tH1\n55398\t27141\tZimmerman\tMN\tSherburne County\tH1\n56304\t27141\tSaint cloud\tMN\tSherburne County\tH1\n55319\t27141\tClear lake\tMN\tSherburne County\tH1\n55371\t27141\tPrinceton\tMN\tSherburne County\tH1\n56329\t27141\tFoley\tMN\tSherburne County\tH1\n55377\t27141\tSantiago\tMN\tSherburne County\tH1\n55312\t27143\tBrownton\tMN\tSibley County\tH1\n55366\t27143\tNew auburn\tMN\tSibley County\tH1\n55339\t27143\tHamburg\tMN\tSibley County\tH1\n55338\t27143\tGreen isle\tMN\tSibley County\tH1\n56054\t27143\tLafayette\tMN\tSibley County\tH1\n55335\t27143\tGibbon\tMN\tSibley County\tH1\n56011\t27143\tBelle plaine\tMN\tSibley County\tH1\n55307\t27143\tArlington\tMN\tSibley County\tH1\n56058\t27143\tLe sueur\tMN\tSibley County\tH1\n55336\t27143\tGlencoe\tMN\tSibley County\tH1\n55396\t27143\tWinthrop\tMN\tSibley County\tH1\n55385\t27143\tStewart\tMN\tSibley County\tH1\n55334\t27143\tGaylord\tMN\tSibley County\tH1\n55332\t27143\tFairfax\tMN\tSibley County\tH1\n56044\t27143\tHenderson\tMN\tSibley County\tH1\n55314\t27143\tBuffalo lake\tMN\tSibley County\tH1\n55353\t27145\tKimball\tMN\tStearns County\tH1\n56312\t27145\tBelgrade\tMN\tStearns County\tH1\n56352\t27145\tMelrose\tMN\tStearns County\tH1\n56362\t27145\tPaynesville\tMN\tStearns County\tH1\n56302\t27145\tSaint cloud\tMN\tStearns County\tH1\n56316\t27145\tBrooten\tMN\tStearns County\tH1\n56307\t27145\tAlbany\tMN\tStearns County\tH1\n55389\t27145\tWatkins\tMN\tStearns County\tH1\n56371\t27145\tRoscoe\tMN\tStearns County\tH1\n56399\t27145\tSaint cloud\tMN\tStearns County\tH1\n56335\t27145\tGreenwald\tMN\tStearns County\tH1\n56398\t27145\tSaint cloud\tMN\tStearns County\tH1\n56310\t27145\tAvon\tMN\tStearns County\tH1\n56336\t27145\tGrey eagle\tMN\tStearns County\tH1\n56368\t27145\tRichmond\tMN\tStearns County\tH1\n56314\t27145\tBowlus\tMN\tStearns County\tH1\n55382\t27145\tSouth haven\tMN\tStearns County\tH1\n56321\t27145\tCollegeville\tMN\tStearns County\tH1\n55329\t27145\tEden valley\tMN\tStearns County\tH1\n56303\t27145\tSaint cloud\tMN\tStearns County\tH1\n56377\t27145\tSartell\tMN\tStearns County\tH1\n56367\t27145\tRice\tMN\tStearns County\tH1\n56374\t27145\tSaint joseph\tMN\tStearns County\tH1\n56331\t27145\tFreeport\tMN\tStearns County\tH1\n56375\t27145\tSaint stephen\tMN\tStearns County\tH1\n55320\t27145\tClearwater\tMN\tStearns County\tH1\n56378\t27145\tSauk centre\tMN\tStearns County\tH1\n56301\t27145\tSaint cloud\tMN\tStearns County\tH1\n56387\t27145\tWaite park\tMN\tStearns County\tH1\n56395\t27145\tSaint cloud\tMN\tStearns County\tH1\n56320\t27145\tCold spring\tMN\tStearns County\tH1\n56340\t27145\tHoldingford\tMN\tStearns County\tH1\n56389\t27145\tWest union\tMN\tStearns County\tH1\n56385\t27145\tVillard\tMN\tStearns County\tH1\n56393\t27145\tSaint cloud\tMN\tStearns County\tH1\n56369\t27145\tRockville\tMN\tStearns County\tH1\n56325\t27145\tElrosa\tMN\tStearns County\tH1\n56376\t27145\tSaint martin\tMN\tStearns County\tH1\n56356\t27145\tNew munich\tMN\tStearns County\tH1\n55060\t27147\tOwatonna\tMN\tSteele County\tH1\n55924\t27147\tClaremont\tMN\tSteele County\tH1\n55049\t27147\tMedford\tMN\tSteele County\tH1\n55946\t27147\tKenyon\tMN\tSteele County\tH1\n55917\t27147\tBlooming prairie\tMN\tSteele County\tH1\n55985\t27147\tWest concord\tMN\tSteele County\tH1\n56026\t27147\tEllendale\tMN\tSteele County\tH1\n56046\t27147\tHope\tMN\tSteele County\tH1\n56093\t27147\tWaseca\tMN\tSteele County\tH1\n56072\t27147\tNew richland\tMN\tSteele County\tH1\n56042\t27147\tHartland\tMN\tSteele County\tH1\n55021\t27147\tFaribault\tMN\tSteele County\tH1\n55052\t27147\tMorristown\tMN\tSteele County\tH1\n56323\t27149\tCyrus\tMN\tStevens County\tH1\n56343\t27149\tKensington\tMN\tStevens County\tH1\n56227\t27149\tCorrell\tMN\tStevens County\tH1\n56267\t27149\tMorris\tMN\tStevens County\tH1\n56248\t27149\tHerman\tMN\tStevens County\tH1\n56235\t27149\tDonnelly\tMN\tStevens County\tH1\n56207\t27149\tAlberta\tMN\tStevens County\tH1\n56244\t27149\tHancock\tMN\tStevens County\tH1\n56221\t27149\tChokio\tMN\tStevens County\tH1\n56226\t27151\tClontarf\tMN\tSwift County\tH1\n56231\t27151\tDanvers\tMN\tSwift County\tH1\n56227\t27151\tCorrell\tMN\tSwift County\tH1\n56289\t27151\tSunburg\tMN\tSwift County\tH1\n56252\t27151\tKerkhoven\tMN\tSwift County\tH1\n56208\t27151\tAppleton\tMN\tSwift County\tH1\n56262\t27151\tMilan\tMN\tSwift County\tH1\n56271\t27151\tMurdock\tMN\tSwift County\tH1\n56249\t27151\tHolloway\tMN\tSwift County\tH1\n56215\t27151\tBenson\tMN\tSwift County\tH1\n56244\t27151\tHancock\tMN\tSwift County\tH1\n56481\t27153\tVerndale\tMN\tTodd County\tH1\n56347\t27153\tLong prairie\tMN\tTodd County\tH1\n56336\t27153\tGrey eagle\tMN\tTodd County\tH1\n56437\t27153\tBertha\tMN\tTodd County\tH1\n56479\t27153\tStaples\tMN\tTodd County\tH1\n56438\t27153\tBrowerville\tMN\tTodd County\tH1\n56443\t27153\tCushing\tMN\tTodd County\tH1\n56319\t27153\tCarlos\tMN\tTodd County\tH1\n56453\t27153\tHewitt\tMN\tTodd County\tH1\n56360\t27153\tOsakis\t
